vi "UI Message Teststand Event Callback.vi"(4 "GUI.lvlib:Auto UI.lvlib:Auto UI.lvclass":refnum<class "Auto UI.lvclass">, 5 "Event Data":cluster{"uiMsg":refnum<k7>, "cancel":bool}, 6 "Control Ref":refnum<k7>, 7 "Event Common Data":T1) -> (1 "Event Data Out":cluster{"cancel":bool})   [LabVIEW 2023, in "GUI.lvlib" / "Auto UI.lvlib" / "Auto UI.lvclass"]
uses:
  Auto UI.lvclass
  <vilib>/ActorFramework/Actor/Actor.lvclass/Actor.ctl
  Main/Main Messages/MenuBar Visable Msg/MenuBar Visable Msg.lvclass/MenuBar Visable Msg.ctl
  <vilib>/ActorFramework/Message Enqueuer/Message Enqueuer.lvclass/Message Enqueuer.ctl
  Auto UI.lvclass/Auto UI.ctl
  <vilib>/ActorFramework/Message Enqueuer/Enqueue.vi
  Main/Main Messages/MenuBar Visable Msg/MenuBar Visable Msg.lvclass
  <vilib>/ActorFramework/Message Priority Queue/Priority Enqueue.vi
  <vilib>/ActorFramework/Actor/Actor.lvclass
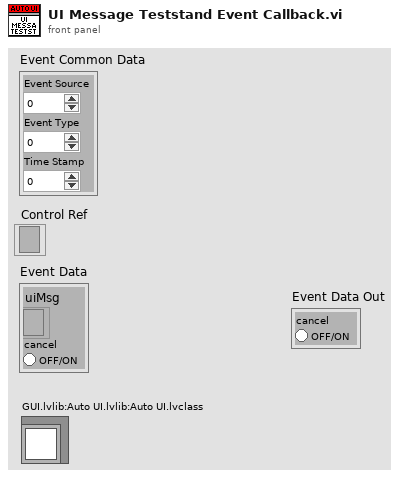
[diagram p1: front panel]
types:
  T1 = cluster{"Event Source":i32, "Event Type":u32, "Time Stamp":u32}
  T2 = enum8{"Enabled", "Disabled", "Disabled and Grayed Out"}
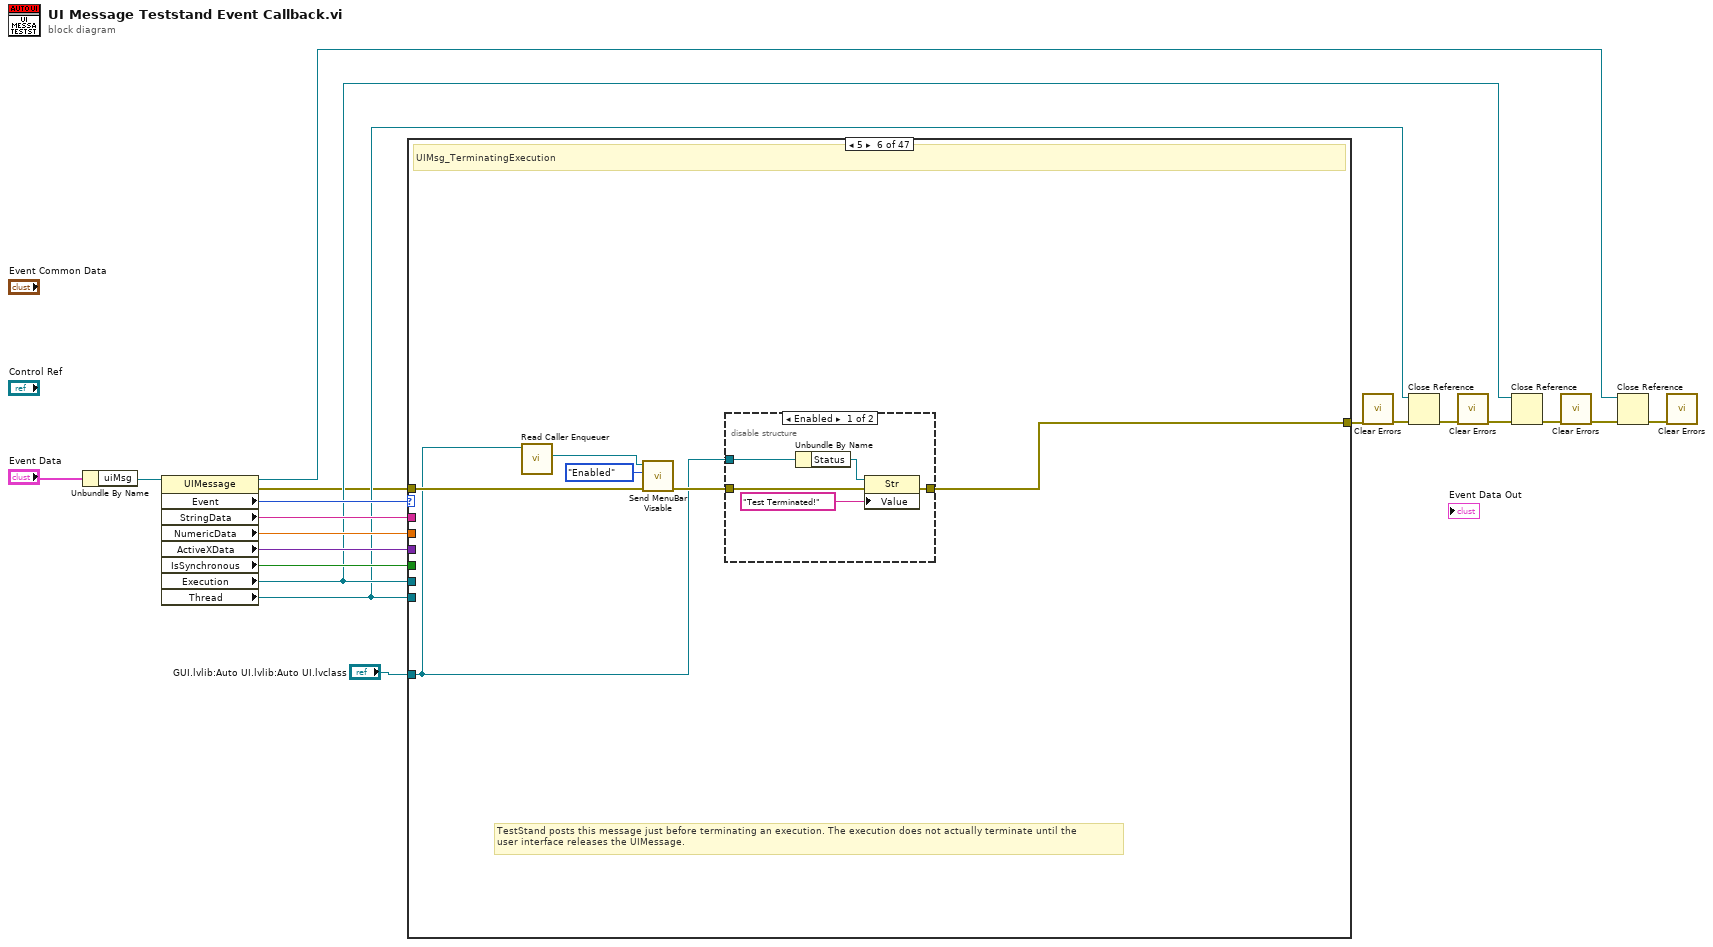
[diagram p0: block diagram]
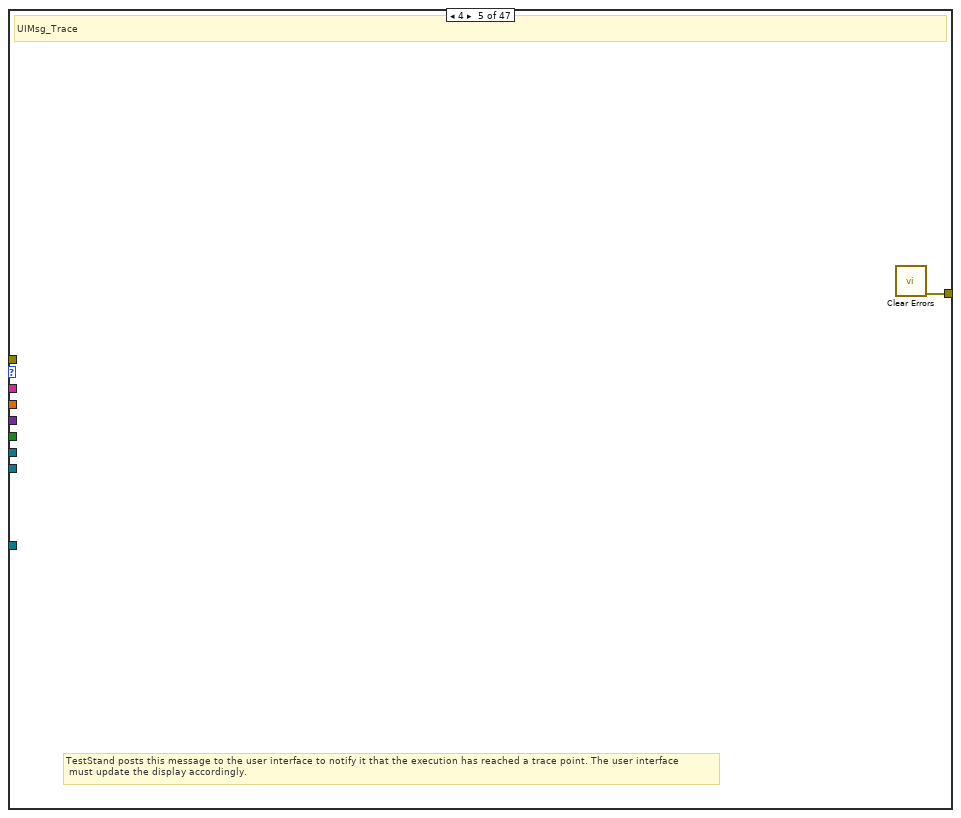
[diagram p6: hidden frame]
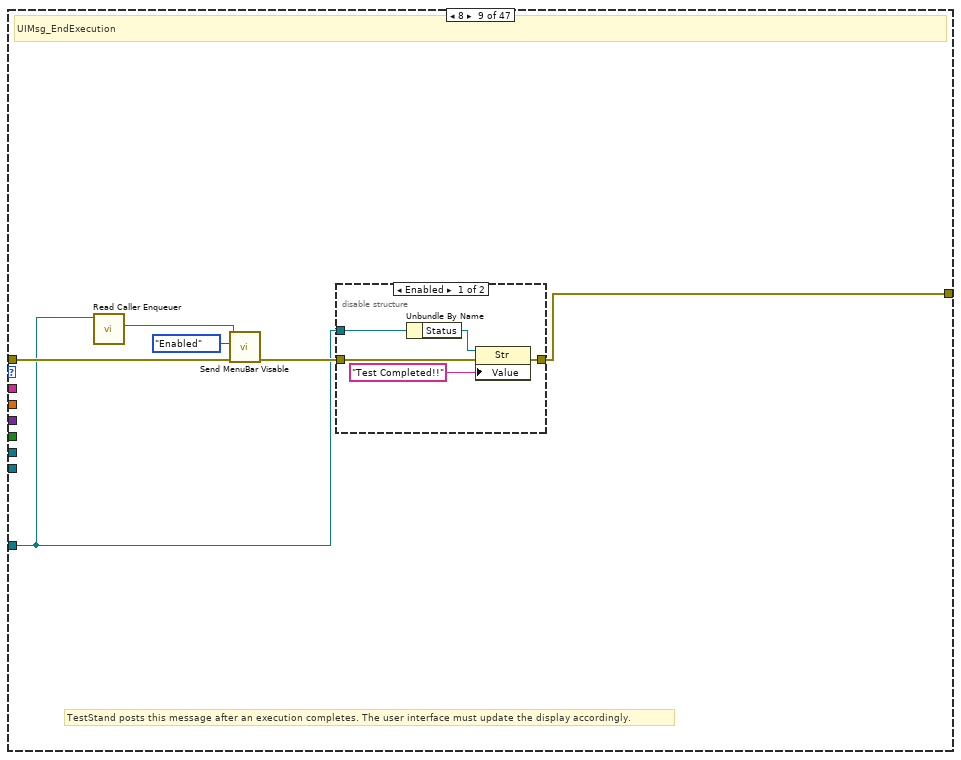
[diagram p10: hidden frame]
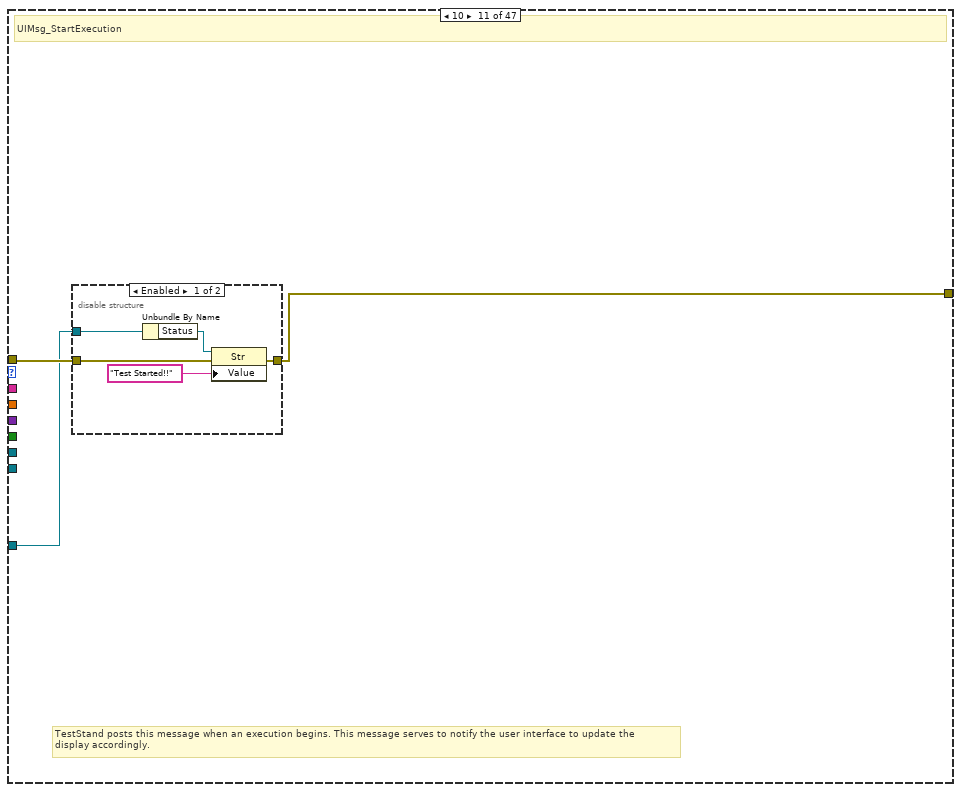
[diagram p13: hidden frame]
diagram:
  n1 = Unbundle By Name("Event Data") -> ("uiMsg"=w14:refnum<k7>)
  n2 = property class="UIMessage"(reference=w14) -> (reference out=w13:refnum<k7>, error out=w1:errorcluster, "Event"=w15:i32, "StringData"=w19:string, "NumericData"=w18:dbl, "ActiveXData"=w17:variant, "IsSynchronous"=w16:bool, "Execution"=w6:refnum<k7>, "Thread"=w4:refnum<k7>)  [unwired: 1 in]
  n3 = case shown="5" w15 {
    tunnel: w19 -> [_ _ _ _ _ _ _ _ _ _ _ _ _ _ _ _ _ _ _ _ _ _ _ _ _ _ _ _ _ _ _ _ _ _ _ _ _ _ _ _ _ _ _ _ _ _ w56]
    tunnel: w18 -> [_ _ _ _ _ _ _ _ _ _ _ _ _ _ _ _ _ _ _ _ _ _ _ _ _ _ _ _ _ _ _ _ _ _ _ _ _ _ _ _ _ _ _ _ _ _ _]
    tunnel: w17 -> [_ _ _ _ _ _ _ _ _ _ _ _ _ _ _ _ _ _ _ _ _ _ _ _ _ _ _ _ _ _ _ _ _ _ _ _ _ _ _ _ _ _ _ _ _ _ _]
    tunnel: w4 -> [_ _ _ _ _ _ _ _ _ _ _ _ _ _ _ _ _ _ _ _ _ _ _ _ _ _ _ _ _ _ _ _ _ _ _ _ _ _ _ _ _ _ _ _ _ _ _]
    tunnel: w6 -> [_ _ _ _ _ _ _ _ _ _ _ _ _ _ _ _ _ _ _ _ _ _ _ _ _ _ _ _ _ _ _ _ _ _ _ _ _ _ _ _ _ _ _ _ _ _ _]
    tunnel: w16 -> [_ _ _ _ _ _ _ _ _ _ _ _ _ _ _ _ _ _ _ _ _ _ _ _ _ _ _ _ _ _ _ _ _ _ _ _ _ _ _ _ _ _ _ _ _ _ _]
    tunnel: [_ _ _ _ w20 w26 _ _ w38 _ w45 _ _ _ _ _ _ _ _ _ _ _ _ _ _ _ _ _ _ _ _ _ _ _ _ _ _ _ _ _ _ _ _ _ _ _ w54] -> w7
    tunnel: "GUI.lvlib:Auto UI.lvlib:Auto UI.lvclass" -> [_ _ _ _ _ w22 _ _ w35 _ w46 _ _ _ _ _ _ _ _ _ _ _ _ _ _ _ _ _ _ _ _ _ _ _ _ _ _ _ _ _ _ _ _ _ _ _ w58]
    tunnel: w1 -> [_ _ _ _ _ w25 _ _ w36 _ w47 _ _ _ _ _ _ _ _ _ _ _ _ _ _ _ _ _ _ _ _ _ _ _ _ _ _ _ _ _ _ _ _ _ _ _ w55]
    frame 0, Default {
    }
    frame 1 {
      # "TestStand posts this message to the user interface to notify it that the execution suspended in response to a user request. \nThe user interface must update the display accordingly."
      # "UIMsg_BreakOnUserRequest"
    }
    frame 2 {
      # "TestStand posts this message to the user interface to notify it that the execution has suspended. The user interface \nmust update the display accordingly."
      # "UIMsg_BreakOnBreakpoint"
    }
    frame 3 {
      # "TestStand posts this message to the user interface to notify it that a run-time error has been encountered in the execution.\n The user interface must update the display accordingly.Note  The engine posts this event only when you select Show \nDialog from the On Run-Time Error ring control on the Execution tab of the Station Options dialog box. A user interface \ntypically calls the Engine.DisplayRunTimeErrorDialogEx method."
      # "UIMsg_BreakOnRunTimeError"
    }
    frame 4 {
      # "TestStand posts this message to the user interface to notify it that the execution has reached a trace point. The user interface\n must update the display accordingly."
      # "UIMsg_Trace"
      n4 = call <vilib>:"Clear Errors.vi"() -> ("error out"=w20:errorcluster)  [unwired: 6 in, 1 out]
    }
    frame 5 {
      # "TestStand posts this message just before terminating an execution. The execution does not actually terminate until the \nuser interface releases the UIMessage."
      # "UIMsg_TerminatingExecution"
      n5 = call <vilib>:"Read Caller Enqueuer.vi"("Actor"=w22) -> ("Caller Enqueuer"=w21:refnum<class "Message Enqueuer.lvclass">)  [unwired: 10 in]
      n6 = call "Send MenuBar Visable.vi"("error in (no error)"=w25, "Disabled"=T2."Enabled", "Message Enqueuer"=w21) -> ("error out"=w24:errorcluster)  [unwired: 7 in, 1 out]
      n7 = disable-structure shown="Enabled" {
        disable-tunnel: w22 -> [w30 _]
        disable-tunnel: w24 -> [w29 w32]
        disable-tunnel: [w28 w32] -> w26
        frame Enabled {
          n8 = Unbundle By Name(w30) -> ("Status"=w31:refnum<vi>)
          n9 = property class="Str"(reference=w31, error in=w29, "Value"="Test Terminated!") -> (error out=w28:errorcluster)  [unwired: 1 out]
        }
        frame Disabled {
        }
      }
    }
    frame 6 {
      # "TestStand posts this message just before aborting an execution. TestStand does not actually abort execution until the \nuser interface releases the UIMessage."
      # "UIMsg_AbortingExecution"
    }
    frame 7 {
      # "TestStand posts this message just before killing the threads in an execution. TestStand does not actually kill the threads \nuntil the user interface releases the UIMessage."
      # "UIMsg_KillingExecutionThreads"
    }
    frame 8 {
      # "TestStand posts this message after an execution completes. The user interface must update the display accordingly."
      # "UIMsg_EndExecution"
      n10 = call <vilib>:"Read Caller Enqueuer.vi"("Actor"=w35) -> ("Caller Enqueuer"=w34:refnum<class "Message Enqueuer.lvclass">)  [unwired: 10 in]
      n11 = call "Send MenuBar Visable.vi"("error in (no error)"=w36, "Disabled"=T2."Enabled", "Message Enqueuer"=w34) -> ("error out"=w37:errorcluster)  [unwired: 7 in, 1 out]
      n12 = disable-structure shown="Enabled" {
        disable-tunnel: w35 -> [w42 _]
        disable-tunnel: w37 -> [w41 w44]
        disable-tunnel: [w40 w44] -> w38
        frame Enabled {
          n13 = Unbundle By Name(w42) -> ("Status"=w43:refnum<vi>)
          n14 = property class="Str"(reference=w43, error in=w41, "Value"="Test Completed!!") -> (error out=w40:errorcluster)  [unwired: 1 out]
        }
        frame Disabled {
        }
      }
    }
    frame 9 {
      # "TestStand posts this message when a shutdown completes. If this is not the final shutdown, the user interface can continue\n to load and execute sequences."
      # "UIMsg_ShutDownComplete"
    }
    frame 10 {
      # "TestStand posts this message when an execution begins. This message serves to notify the user interface to update the \ndisplay accordingly."
      # "UIMsg_StartExecution"
      n15 = disable-structure shown="Enabled" {
        disable-tunnel: w46 -> [w51 _]
        disable-tunnel: w47 -> [w50 w53]
        disable-tunnel: [w49 w53] -> w45
        frame Enabled {
          n16 = Unbundle By Name(w51) -> ("Status"=w52:refnum<vi>)
          n17 = property class="Str"(reference=w52, error in=w50, "Value"="Test Started!!") -> (error out=w49:errorcluster)  [unwired: 1 out]
        }
        frame Disabled {
        }
      }
    }
    frame 11 {
      # "TestStand step modules post this message to the user interface to notify it to update the progress indicator associated \nwith an execution. The activeXDataParam parameter specifies an execution. The numericDataParam parameter specifies \na value from 0 to 100 that indicates the percentage of progress the current execution reports. This value indicates the progress \nof operations for which the execution chooses to report the amount of progress. The value does not necessarily reflect the \nprogress of the execution as a whole."
      # "UIMsg_ProgressPercent"
    }
    frame 12 {
      # "TestStand step modules post this message to the user interface to notify it to update the progress message associated\nwith an execution. The activeXDataParam parameter specifies an execution. The stringDataParam parameter specifies \na progress message."
      # "UIMsg_ProgressText"
    }
    frame 13 {
      # "TestStand posts this message whenever an interactive execution begins."
      # "UIMsg_StartInteractiveExecution"
    }
    frame 14 {
      # "TestStand posts this message whenever an interactive execution ends."
      # "UIMsg_EndInteractiveExecution"
    }
    frame 15 {
      # "TestStand posts this message just before terminating an interactive execution. The interactive execution does not actually \nterminate until the user interface message is released."
      # "UIMsg_TerminatingInteractiveExecution"
    }
    frame 16 {
      # "TestStand posts this message to notify the user interface to update the display when a pending termination is cancelled."
      # "UIMsg_TerminationCancelled"
    }
    frame 17 {
      # "TestStand posts this message when an execution resumes after being suspended at a breakpoint. The execution resumes \nwhen the user interface message is released."
      # "UIMsg_ResumeFromBreak"
    }
    frame 18 {
      # "TestStand posts this message when it begins using a sequence file. TestStand specifies the file in the UIMessage.\nActiveXData property."
      # "UIMsg_StartFileExecution"
    }
    frame 19 {
      # "TestStand posts this message when the execution finishes using a sequence file. TestStand specifies the file in the \nUIMessage.ActiveXData property."
      # "UIMsg_EndFileExecution"
    }
    frame 20 {
      # "TestStand posts this message to notify the user interface that the user cancelled a pending shutdown."
      # "UIMsg_ShutDownCancelled"
    }
    frame 21 {
      # "TestStand posts this message to notify the user interface that the decimal point localization setting has changed \nin the system setting for the operating system or in the StationOptions.UseLocalizedDecimalPoint setting. When \na user interface receives this message, it should refresh any values it displays that these changes might affect."
      # "UIMsg_LocalizationSettingChanged"
    }
    frame 22 {
      # "Post this message to the user interface to instruct it to open a file in a window. If the file or execution is already open, \nthe application brings the file to the front. A file can be specified by a pathname in the stringDataParam parameter or \nby a PropertyObjectFile object in the activeXDataParam parameter. An execution can be specified by an Execution \nobject in the activeXDataParam parameter. A list of files and/or executions can be specified by an array of references to \nPropertyObjectFile and Execution objects in the activeXDataParam parameter. For sequence files, the stringDataParam \nparameter can also contain a '|' separator followed by the name of a sequence to display. If you specify the sequence \nfile in the activeXDataParam parameter, you can specify just the sequence name in the stringDataParam parameter. \nThis constant does not support opening workspace files."
      # "UIMsg_OpenWindows"
    }
    frame 23 {
      # "Post this message to the user interface to instruct it to tile the windows the activeXDataParam parameter specifies. Use an \narray of ActiveX reference objects that reference a PropertyObjectFile or an Execution for the activeXDataParam parameter. \nThe user interface tiles the windows that correspond to the objects in the array. To tile all windows, pass a NULL reference \nfor the activeXDataParam parameter or use the Nothing keyword if you are using the ActiveX/COM Adapter."
      # "UIMsg_TileWindows"
    }
    frame 24 {
      # "Post this message to the user interface to instruct it to cascade the windows the activeXDataParam parameter specifies. \nUse an array of ActiveX reference objects that reference a PropertyObjectFile or an Execution for the activeXDataParam \nparameter. The user interface cascades the windows that correspond to the objects in the array. To cascade all windows, \npass a NULL reference for the activeXDataParam parameter or use the Nothing keyword if you are using the ActiveX/COM \nAdapter."
      # "UIMsg_CascadeWindows"
    }
    frame 25 {
      # "The TestStand Engine posts this message to the user interface whenever you update the report of an execution. This allows the \nuser interface to refresh the Report view if it is showing."
      # "UIMsg_ReportChanged"
    }
    frame 26 {
      # "Post this message to the user interface to instruct it to close a window or windows that display a PropertyObjectFile or an \nexecution. Specify the window by passing a PropertyObjectFile or Execution reference for the activeXDataParam parameter, \nor specify several windows by passing an ActiveX reference array of such objects for the activeXDataParam parameter. \nPass a NULL reference, or use the Nothing keyword if you are using the ActiveX/COM Adapter, to close all currently open \ndocument windows in the user interface."
      # "UIMsg_CloseWindows"
    }
    frame 27 {
      # "Post this message to the user interface to instruct it to refresh the data it displays for the corresponding PropertyObjectFile \nor SequenceContext you pass for the activeXDataParam parameter. Pass a single reference or an ActiveX array of references\nusing the activeXDataParam parameter to specify which window or windows to refresh. Pass a SequenceContext object to \nrefresh the values for the steps which the user interface displays for that execution. Pass NULL for the activeXDataParam \nparameter to refresh the displays for all the files and executions. The Overriding SequenceFilePostStepFailure Callback and \nthe Overriding SequenceFilePostStepRuntimeError Callback examples located in the <TestStand Public>\\Examples\\Modifying \nProcess Models\\Overriding Engine Callbacks directory demonstrate how to use this UIMessage."
      # "UIMsg_RefreshWindows"
    }
    frame 28 {
      # "An Execution object posts this message when a client changes the value of the Execution.ClientFile property. \nThe UIMessage.Execution property references the Execution that sends the message."
      # "UIMsg_ClientFileChanged"
    }
    frame 29 {
      # "Post this message when you want the user interface to display the current contents of the execution report."
      # "UIMsg_DisplayReport"
    }
    frame 30 {
      # "TestStand process models post this message to the user interface before performing initialization prior to testing. \nThe numericDataParam parameter specifies the test-socket index. The activeXDataParam parameter contains a \nreference to the sequence context for the process model sequence file that posts the message."
      # "UIMsg_ModelState_Initializing"
    }
    frame 31 {
      # "TestStand process models post this message to the user interface before waiting for an action to occur, such as the user \nentering a serial number in response to a prompt. The numericDataParam parameter specifies the test-socket index. \nThe activeXDataParam parameter contains a reference to the sequence context for the process model sequence file that \nposts the message."
      # "UIMsg_ModelState_Waiting"
    }
    frame 32 {
      # "Test Socket"
      # "UUT Serail Number"
      # "TestStand process models post this message to the user interface after identifying the serial number for a unit under test (UUT)\n or batch of UUTs. The stringDataParam parameter specifies the UUT serial number unless the execution is a batch controller. \nIf the execution is a batch controller, the stringDataParam parameter specifies the batch serial number. The numericDataParam \nparameter specifies the test-socket index. The activeXDataParam parameter contains a reference to the sequence context for \nthe process model sequence file that posts the message."
      # "UIMsg_ModelState_Identified"
    }
    frame 33 {
      # "TestStand process models post this message to the user interface prior to calling MainSequence in the client sequence file. \nThe numericDataParam parameter specifies the test-socket index. The activeXDataParam parameter contains a reference to \nthe sequence context for the process model sequence file that posts the message."
      # "UIMsg_ModelState_BeginTesting"
    }
    frame 34 {
      # "If the Onfail to Cleanup"
      # "TestStand process models post this message to the user interface after the MainSequence in the client sequence file returns \ncontrol to the model. If the execution is not a batch controller or a parallel controller, the stringDataParam parameter specifies \nthe UUT result status. If the execution is a batch controller or a parallel controller, the value of the stringDataParam parameter \nspecifies the overall status of the controlling execution, which by default can be Passed, Failed, Error, Terminated, or Aborted. \nThe numericDataParam parameter specifies the test-socket index. The activeXDataParam parameter contains a reference to \nthe sequence context for the process model sequence file that posts the message."
      # "UIMsg_ModelState_TestingComplete"
    }
    frame 35 {
      # "TestStand process models post this message to the user interface after generating the report and logging the data for a \nclient sequence file. The numericDataParam parameter specifies the test-socket index. The activeXDataParam parameter \ncontains a reference to the sequence context for the process model sequence file that posts the message."
      # "UIMsg_ModelState_PostProcessingComplete"
    }
    frame 36 {
      # "TestStand Batch process models post this message to the user interface after setting the enabled state of a \ntest-socket execution. The value of the stringDataParam parameter is True if the socket is enabled and False if the \nsocket is disabled. The numericDataParam parameter specifies the test-socket index. The activeXDataParam parameter \ncontains a reference to the sequence context for the process model sequence file that posts the \nmessage."
      # "UIMsg_ModelState_EnabledStateSet"
    }
    frame 37 {
      # "The TestStand Engine posts this message to the user interface whenever you change the location of the report."
      # "UIMsg_ReportLocationChanged"
    }
    frame 38 {
      # "The Locations.GotoLocation method posts this message to the user interface to instruct the user interface to select the \nLocations passed in as the activeXDataParam parameter."
      # "UIMsg_GotoLocation"
    }
    frame 39 {
      # "Post this message to the sequence editor to instruct the sequence editor to push an undo item onto an UndoStack. \nAn undo item is a COM object that implements the UndoItem interface. You pass the undo item as the activeXDataParam \nparameter. The sequence editor uses the UndoItem.EditedFile property to determine which UndoStack to push the undo \nitem onto. Send this message synchronously to determine which UndoStack the sequence editor placed the undo item \nonto immediately after the call to the PostUIMessage method returns by checking the UndoItem.UndoStack property."
      # "UIMsg_PushUndoItem"
    }
    frame 40 {
      # "TestStand posts this message at periodic intervals when it holds references to output messages that calls to the OutputMessage.\nPost method queue. TestStand transfers the queued messages to an OutputMessages collection attached to the UIMessage.\nActiveXData property for this event. Ensure that an application that processes output messages copies the output message \nreferences from the collection in UIMessage.ActiveXData to a private OutputMessages collection by passing the private collection\n to the OutputMessages.CopyMessagesToCollection method. An application calls the Engine.NewOutputMessages method to \ncreate a private OutputMessage collection. TestStand generates this event only if the Engine.OutputMessagesEnabled property\n is True. Because there can be more than one handler for this event, ensure that the application does not modify the \nOutputMessages collection the UIMessage.ActiveXData property holds."
      # "UIMsg_OutputMessages"
    }
    frame 41 {
      # "TestStand posts this message to the user interface to notify it that the type palette file list has changed. The user interface must \nupdate its display accordingly. This event occurs after calling the Engine.UnloadTypePaletteFiles, Engine.LoadTypePaletteFilesEx, \nand Engine.SetTypePaletteFileList methods."
      # "UIMsg_TypePaletteFileListChanged"
    }
    frame 42 {
      # "An execution posts this message when it attempts to terminate and every thread in the execution uses a value of \nThreadTerminationOptions_Prompt for the Thread.TerminationOption property. A user interface typically handles this \nevent by prompting users to terminate all threads. If the user chooses to terminate all threads, the user interface calls the \nExecution.OverrideNonTerminatableThreads property to signal the threads that use a value of \nThreadTerminationOptions_Prompt for the Thread.TerminationOption property to stop running."
      # "UIMsg_NonTerminatableThreadsArePreventingTermination"
    }
    frame 43 {
      # "TestStand process models post this message to the user interface before generating the report and logging the data for \na client sequence file. The numericDataParam parameter specifies the test-socket index. The activeXDataParam parameter \ncontains a reference to the sequence context for the process model sequence file that posts the message."
      # "UIMsg_ModelState_PostProcessing"
    }
    frame 44 {
      # "The TestStand Engine posts this message when the content or an active report changes for the Reports collection of an execution. \nIf the active report changes, the activeXDataParam parameter contains a reference to the previously active report."
      # "UIMsg_ReportCollectionChanged"
    }
    frame 45 {
      # "TestStand posts this message to the user interface to notify the user interface that the execution has encountered a run-time error. \nThe user interface can alter the error, for example, by adding contextual information to the error message."
      # "UIMsg_RuntimeError"
    }
    frame 10000 {
      # "UI Auto Status Update"
      # "Codes for all user-defined messages must be greater than or equal to the value of this constant. Define and use event codes \ngreater than UIMsg_UserMessageBase only when you can ensure that the event code does not conflict with event codes \nfor messages that other custom TestStand components, such as add-on products, define. National Instruments recommends \nusing the Engine.RegisterUIMessage method to obtain an event code for a message to guarantee that the code is unique for \nthe lifetime of the engine. Components that generate and process the message call this method, which returns the previously \nassigned message code if the message is already assigned."
      # "UIMsg_UserMessageBase"
      n18 = Unbundle By Name(w58) -> ("Status"=w57:refnum<vi>)
      n19 = property class="Str"(reference=w57, error in=w55, "Value"=w56) -> (error out=w54:errorcluster)  [unwired: 1 out]
    }
  }
  n20 = call <vilib>:"Clear Errors.vi"("error in (no error)"=w7) -> ("error out"=w8:errorcluster)  [unwired: 5 in, 1 out]
  n21 = Close Reference(reference=w4, error in (no error)=w8) -> (error out=w5:errorcluster)
  n22 = call <vilib>:"Clear Errors.vi"("error in (no error)"=w5) -> ("error out"=w9:errorcluster)  [unwired: 5 in, 1 out]
  n23 = Close Reference(reference=w6, error in (no error)=w9) -> (error out=w11:errorcluster)
  n24 = call <vilib>:"Clear Errors.vi"("error in (no error)"=w11) -> ("error out"=w10:errorcluster)  [unwired: 5 in, 1 out]
  n25 = Close Reference(reference=w13, error in (no error)=w10) -> (error out=w12:errorcluster)
  n26 = call <vilib>:"Clear Errors.vi"("error in (no error)"=w12) -> ()  [unwired: 5 in, 2 out]
